vi "GetExposureStatus.vi"(0 "Readout Time":dbl, 4 "% Complete Caption":string, 6 "Previous % Complete Value":dbl, 7 "Exposure Time":dbl, 8 "Mode #":dbl, 9 "Initial Time":dbl) -> (1 "Exp time left":dbl, 2 "Readout left":dbl, 3 "% Exposed":dbl, 5 "% Complete":dbl)   [LabVIEW 2015]
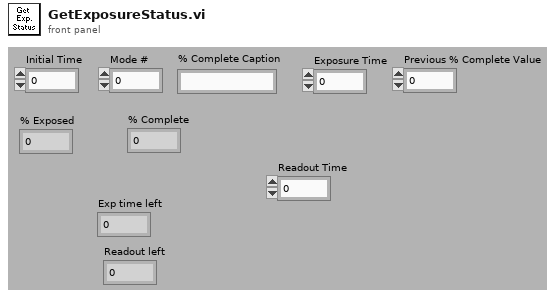
[diagram p1: front panel]
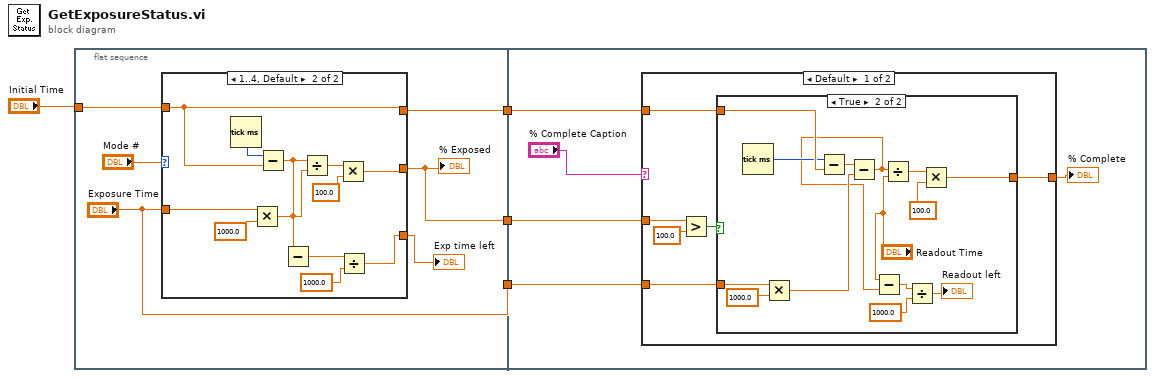
[diagram p0: block diagram]
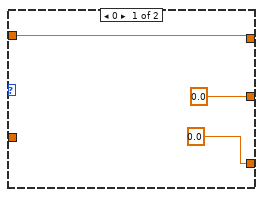
[diagram p2: hidden frame]
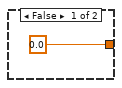
[diagram p3: hidden frame]
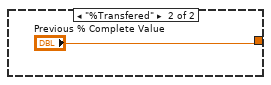
[diagram p4: hidden frame]
diagram:
  n1 = flat-sequence {
    tunnel: "Initial Time" -> [w9]
    tunnel: [w8] -> w3
    tunnel: [w7] -> w2
    tunnel: ["Exposure Time"] -> w1
    tunnel: w3 -> [w28]
    tunnel: w2 -> [w29]
    tunnel: w1 -> [w27]
    frame #0 {
      n2 = case shown="1..4, Default" "Mode #" {
        tunnel: w9 -> [w13 w24]
        tunnel: [w13 w24] -> w8
        tunnel: [0.0 ("% Exposed") w20] -> w7
        tunnel: "Exposure Time" -> [_ w19]
        tunnel: [0.0 w14] -> w5
        frame 0 {
        }
        frame 1..4, Default {
          n3 = Tick Count (ms)() -> (millisecond timer value=w25:u32)
          n4 = Multiply(x=w19, y=1000.0) -> (x*y=w18:dbl)
          n5 = Subtract(x=w25, y=w24) -> (x-y=w17:dbl)
          n6 = Subtract(x=w18, y=w17) -> (x-y=w16:dbl)
          n7 = Divide(x=w17, y=w18) -> (x/y=w22:dbl)
          n8 = Multiply(x=w22, y=100.0) -> (x*y=w20:dbl)
          n9 = Divide(x=w16, y=1000.0) -> (x/y=w14:dbl)
        }
      }
      "% Exposed" <- w7
      "Exp time left" <- w5
    }
    frame #1 {
      n10 = case shown="Default" "% Complete Caption" {
        tunnel: w29 -> [w36 _]
        tunnel: w28 -> [w33 _]
        tunnel: w27 -> [w32 _]
        tunnel: [w31 "Previous % Complete Value"] -> w26
        frame Default {
          n11 = Greater?(x=w36, y=100.0) -> (0:w34:bool)
          n12 = case shown="True" w34 {
            tunnel: w33 -> [_ w51]
            tunnel: [0.0 w48] -> w31
            tunnel: w32 -> [_ w47]
            frame False {
            }
            frame True {
              n13 = Tick Count (ms)() -> (millisecond timer value=w45:u32)
              n14 = Multiply(x=w47, y=1000.0) -> (x*y=w43:dbl)
              n15 = Subtract(x=w45, y=w51) -> (x-y=w44:dbl)
              n16 = Subtract(x=w44, y=w43) -> (x-y=w41:dbl)
              n17 = Subtract(x="Readout Time", y=w41) -> (x-y=w40:dbl)
              n18 = Divide(x=w41, y="Readout Time") -> (x/y=w50:dbl)
              n19 = Divide(x=w40, y=1000.0) -> (x/y=→"Readout left":dbl)
              n20 = Multiply(x=w50, y=100.0) -> (x*y=w48:dbl)
            }
          }
        }
        frame "%Transfered" {
        }
      }
      "% Complete" <- w26
    }
  }
